vi "Append Text HF.vi"(0 "PDF Report IN":T24(xcontrol), 2 "Header or footer":T1={"Start at page"=1, "H/F Alignment"=enum."RIGHT - middle", "Text"="", "Font"={"Name"="Helvetica", "Size"=12.0, "Color"=0, "Style"={"Bold"=FALSE, "Italic"=FALSE, "Underline"=FALSE, "Strikeout"=FALSE}}, "Link"=""}, 11 "error in (no error)":errorcluster, 13 "Position":T6) -> (4 "PDF Report OUT":T24(xcontrol), 15 "error out":errorcluster)   [LabVIEW 2012]
doc: "Appends <B>text</B> in a column header (or footer). You can use this polymorphic VI to append a colomn to a header (or footer). The data type you wire to the <B>Header or footer</B> input determines the polymorphic instance to use.\n\nThe header (or footer) can be divided up into three columns. Each column has the same width. The number of header (or footer) that you add determines the number of columns.\n\n<B>FRANÇAIS</B>\nAjoute du <B>texte</B> dans une colonne d'un en-tête (ou d'un pied de page). Vous pouvez utiliser ce VI polymorphique pour ajouter une colonne à un en-tête (ou un pied de page). Le type de variable que vous reliez au terminal <B>Header or footer</B> détermine l'instance polymorphique à utiliser.\n\nL'en-tête (ou le pied de page) peut être divisé en un maximum de trois colonnes. Chaque colonne a la même largeur. Le nombre d'en-têtes (ou de pieds de page) que vous ajoutez détermine le nombre de colonnes.\n\n\n\nVersion 1.0\nDeveloped by Jean-Marc Simard\nCopyright © 2010, Exaprom Inc.\nAll rights reserved.\nLicense: BSD\n\nWith iTextSharp 4.1.6 (http://itextsharp.sourceforge.net)\nunder Mozilla Public License Version 1.1\n(http://www.mozilla.org/MPL/MPL-1.1.html)"
uses:
  Controls/Header Footer Type.ctl
  Controls/Header footer horiz alignment.ctl
  Controls/Cell Vertical alignment.ctl
  Controls/Page number.ctl
  Controls/Font size.ctl
  Controls/Font color.ctl
  Controls/Font cluster.ctl
  Controls/Header Footer Line.ctl
  Controls/Header Footer cluster.ctl
  C:/Users/MaxCorp/Documents/GitHub/TopView/DLL/itextsharp.dll
  GitHub/TopView/DLL/itextsharp.dll
  Controls/H F Alignment.ctl
  Controls/Header or Footer.ctl
  Controls/PDF Report Xcontrol/PDF Report.xctl
  Controls/Header or Footer  Text cluster.ctl
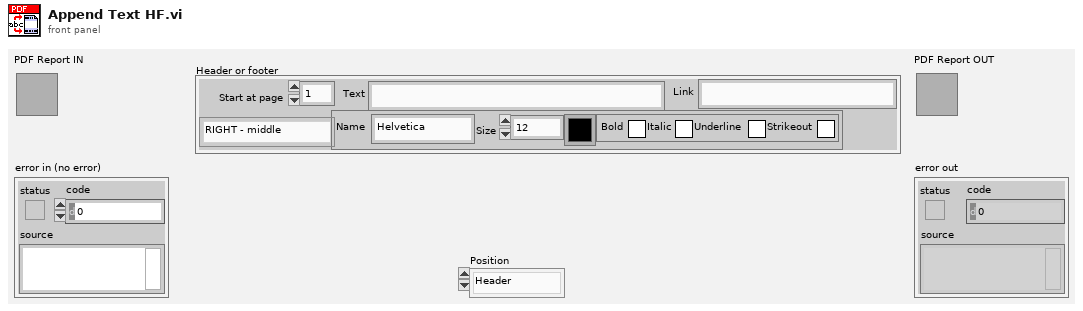
[diagram p1: front panel]
types:
  T1 = typedef "Header or Footer  Text cluster.ctl" = cluster{"Start at page":i32, "H/F Alignment":T2, "Text":string, "Font":T3, "Link":string}
  T2 = typedef "H F Alignment.ctl" = enum16{"LEFT - top", "LEFT - middle", "LEFT - bottom", "CENTER - top", "CENTER - middle", "CENTER - bottom", "RIGHT - top", "RIGHT - middle", "RIGHT - bottom", ""}
  T3 = typedef "Font cluster.ctl" = cluster{"Name":string, "Size":T4, "Color":T5, "Style":cluster{"Bold":bool, "Italic":bool, "Underline":bool, "Strikeout":bool}}
  T4 = typedef "Font size.ctl" = sgl
  T5 = typedef "Font color.ctl" = u32
  T6 = typedef "Header or Footer.ctl" = enum16{"Header", "Footer"}
  T7 = typedef "Unit.ctl" = enum16{"inch", "mm"}
  T8 = typedef "Paragraphe cluster.ctl" = cluster{" Aligment":T9, "Line spacing":T10}
  T9 = typedef "Texte alignement.ctl" = enum16{"Select", "CENTER", "JUSTIFY", "LEFT", "RIGHT"}
  T10 = typedef "Line spacing.ctl" = enum16{"Select", "1.0", "1.5", "2.0"}
  T11 = typedef "Page dimensions.ctl" = cluster{"Start at page":i32, "Orientation":T12, "widht":sgl, "height":sgl, "Margin left":sgl, "Margin right":sgl, "Margin top":sgl, "Margin bottom":sgl}
  T12 = typedef "Page Orientation.ctl" = enum16{"Portrait", "Landscape"}
  T13 = typedef "Image or Table Caption.ctl" = cluster{"Caption":string, "Separator":string, "Position":enum16{"Above", "Below"}}
  T14 = typedef "Header Footer [ ].ctl" = T15[]
  T15 = typedef "Header Footer cluster.ctl" = cluster{"Start page":i32, "Type":T16, "Alignment":T17, "Vertical Alignement":T18, "Image (%)":sgl, "Page #":T19, "Text":string, "Path":string, "Font":T3, "Font refnum":refnum<k24>, "Line":cluster{"Line":T20, "Thickness (points)":sgl, "Colour":T5}}
  T16 = typedef "Header Footer Type.ctl" = enum16{"Select", "Text", "Text + hyperlink", "Page number", "Image", "Image + hyperlink"}
  T17 = typedef "Header footer horiz alignment.ctl" = enum16{"Left", "Center", "Right"}
  T18 = typedef "Cell Vertical alignment.ctl" = enum16{"TOP", "MIDDLE", "BOTTOM"}
  T19 = typedef "Page number.ctl" = cluster{"Text 1":string, "Text 2":string, "Text 3":string}
  T20 = typedef "Header Footer Line.ctl" = enum16{"No line", "Horizontal line"}
  T21 = typedef "Watermark cluster2.ctl" = cluster{"Show? (F)":bool, "Type":enum16{"Image", "Text"}, "Opacity (%)":sgl, "Rotate(°)":sgl, "Position":cluster{"Position":T22, "X":sgl, "Y":sgl}, "Image path":path, "Scaled(%)":sgl, "Image refnum":refnum<k24>, "Text":string, "Font":cluster{"Name":string, "Size":T4, "Color":T5}, "Font refnum":refnum<k24>, "Alignment":T17, "Automatic":bool}
  T22 = typedef "Watermark Position.ctl" = enum16{"Absolute", "Center (page)", "Center (text section)"}
  T23 = typedef "System Fonts.ctl" = cluster{"Font name [ ]":string[], "Font and file names [ ]":cluster{"Font name":string, "File name":string}[]}
  T24 = cluster{"Document":refnum<k24>, "Writer":refnum<k24>, "Default Font":refnum<k24>, "Default Font cluster":T3, "Path":path, "Unit (default = mm)":T7, "Paragraphe cluster":T8, "Pages dimensions [ ]":T11[], "Captions":cluster{"Image":T13, "Image counter":u16, "Table":T13, "Table counter":u16, "Font":T3}, "Header":T14, "Footer":T14, "Watermark ":T21, "Actual VI name":string, "System Fonts":T23}
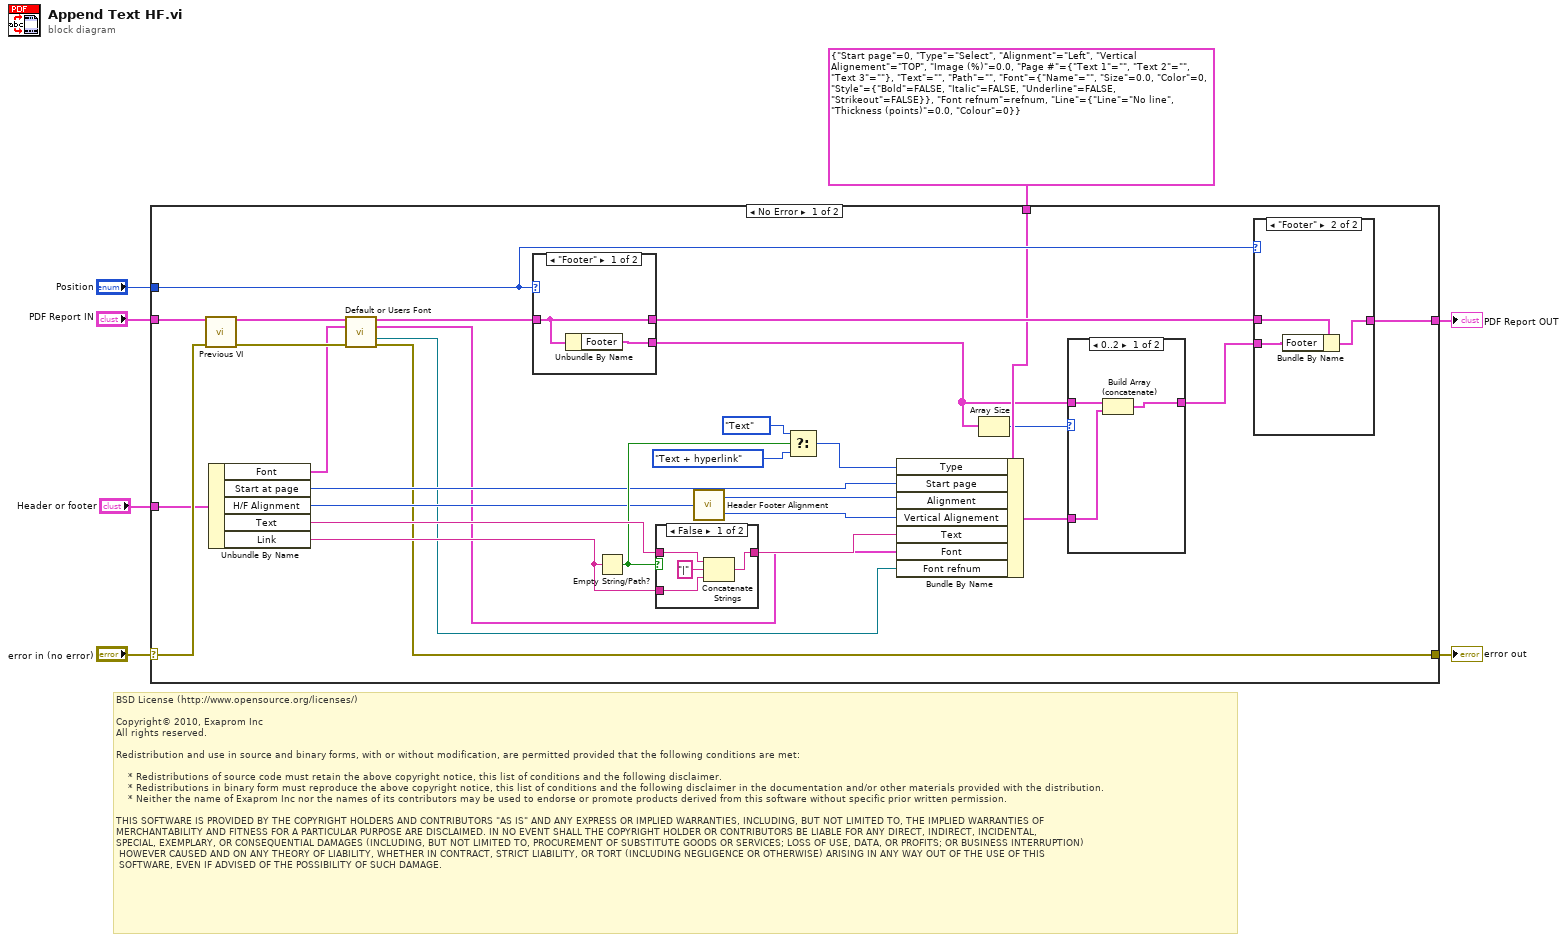
[diagram p0: block diagram]
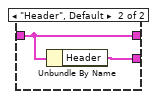
[diagram p4: hidden frame]
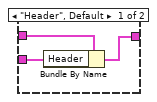
[diagram p5: hidden frame]
diagram:
  # "BSD License (http://www.opensource.org/licenses/)\n\nCopyright© 2010, Exaprom Inc\nAll rights reserved.\n\nRedistribution and use in source and binary forms, with or without modification, are permitted provided that the following conditions are met:\n\n    * Redistributions of source code must retain the above copyright notice, this list of conditions and the following disclaimer.\n    * Redistributions in binary form must reproduce the above copyright notice, this list of conditions and the following disclaimer in the documentation and/or other materials provided with the distribution.\n    * Neither the name of Exaprom Inc nor the names of its contributors may be used to endorse or promote products derived from this software without specific prior written permission.\n\nTHIS SOFTWARE IS PROVIDED BY THE COPYRIGHT HOLDERS AND CONTRIBUTORS \"AS IS\" AND ANY EXPRESS OR IMPLIED WARRANTIES, INCLUDING, BUT NOT LIMITED TO, THE IMPLIED WARRANTIES OF \nMERCHANTABILITY AND FITNESS FOR A PARTICULAR PURPOSE ARE DISCLAIMED. IN NO EVENT SHALL THE COPYRIGHT HOLDER OR CONTRIBUTORS BE LIABLE FOR ANY DIRECT, INDIRECT, INCIDENTAL,\nSPECIAL, EXEMPLARY, OR CONSEQUENTIAL DAMAGES (INCLUDING, BUT NOT LIMITED TO, PROCUREMENT OF SUBSTITUTE GOODS OR SERVICES; LOSS OF USE, DATA, OR PROFITS; OR BUSINESS INTERRUPTION)\n HOWEVER CAUSED AND ON ANY THEORY OF LIABILITY, WHETHER IN CONTRACT, STRICT LIABILITY, OR TORT (INCLUDING NEGLIGENCE OR OTHERWISE) ARISING IN ANY WAY OUT OF THE USE OF THIS\n SOFTWARE, EVEN IF ADVISED OF THE POSSIBILITY OF SUCH DAMAGE."
  n1 = case shown="No Error" "error in (no error)" {
    selector: "error in (no error)" -> [w16 w57]
    tunnel: "PDF Report IN" -> [w17 w56]
    tunnel: "Position" -> [w24 _]
    tunnel: [w36 w56] -> w5
    tunnel: [w10 w57] -> w4
    tunnel: "Header or footer" -> [w15 _]
    tunnel: T15 {"Start page"=0, "Type"=enum."Select", "Alignment"=enum."Left", "Vertical Alignement"=enum."TOP", "Image (%)"=0.0, "Page #"={"Text 1"="", "Text 2"="", "Text 3"=""}, "Text"="", "Path"="", "Font"={"Name"="", "Size"=0.0, "Color"=0, "Style"={"Bold"=FALSE, "Italic"=FALSE, "Underline"=FALSE, "Strikeout"=FALSE}}, "Font refnum"=refnum, "Line"={"Line"=enum."No line", "Thickness (points)"=0.0, "Colour"=0}} ("element") -> [w20 _]
    frame No Error {
      n2 = call "Previous VI.vi"("PDF Report IN"=w17, "error in (no error)"=w16) -> ("PDF Report OUT"=w14:T24, "error out"=w12:errorcluster)  [unwired: 12 out]
      n3 = Unbundle By Name(w15) -> ("Font"=w11:T3, "Start at page"=w26:i32, "H/F Alignment"=w23:T2, "Text"=w31:string, "Link"=w33:string)
      n4 = call "Default or Users Font.vi"("PDF Report"=w14, "Font"=w11, "error in (no error)"=w12) -> ("PDF Report duplicate"=w13:T24, "Font OUT"=w9:T3, "Font Ref"=w8:refnum<k24>, "error out"=w10:errorcluster)  [unwired: 9 out]
      n5 = case shown="\"Footer\"" w24 {
        tunnel: w13 -> [w47 w49]
        tunnel: [w47 w49] -> w35
        tunnel: [w46 w48] -> w18
        frame "Footer" {
          n6 = Unbundle By Name(w47) -> ("Footer"=w46:T14)
        }
        frame "Header", Default {
          n7 = Unbundle By Name(w49) -> ("Header"=w48:T14)
        }
      }
      n8 = Empty String/Path?(string/path=w33) -> (empty?=w30:bool)
      n9 = case shown="False" w30 {
        tunnel: w31 -> [w44 w45]
        tunnel: [w43 w45] -> w32
        tunnel: w33 -> [w41 _]
        frame False {
          n10 = Concatenate Strings(w44, "|" ("string"), w41) -> (w43:string)
        }
        frame True {
        }
      }
      n11 = call "Header Footer Alignment.vi"("H/F Alignment"=w23) -> ("Vertical Alignement"=w21:T18, "Horizontal Alignment"=w22:T17)  [unwired: 2 out]
      n12 = Select(t=Header_Footer_Type."Text" ("Type"), s=w30, f=Header_Footer_Type."Text + hyperlink" ("Type")) -> (s? t:f=w29:T16)
      n13 = Bundle By Name(cluster=w20, "Type"=w29, "Start page"=w26, "Alignment"=w22, "Vertical Alignement"=w21, "Text"=w32, "Font"=w9, "Font refnum"=w8) -> (w34:T15)
      n14 = Array Size(array=w18) -> (size(s)=w19:i32)
      n15 = case shown="0..2" w19 {
        tunnel: w34 -> [w39 _]
        tunnel: [w37 w40] -> w25
        tunnel: w18 -> [w38 w40]
        frame 0..2 {
          n16 = Build Array (concatenate)(w38, w39) -> (w37:T14)
        }
        frame 3.., Default {
        }
      }
      n17 = case shown="\"Footer\"" w24 {
        tunnel: w35 -> [w52 w55]
        tunnel: w25 -> [w50 w53]
        tunnel: [w51 w54] -> w36
        frame "Header", Default {
          n18 = Bundle By Name(cluster=w52, "Header"=w50) -> (w51:T24)
        }
        frame "Footer" {
          n19 = Bundle By Name(cluster=w55, "Footer"=w53) -> (w54:T24)
        }
      }
    }
    frame Error {
    }
  }
  "PDF Report OUT" <- w5
  "error out" <- w4
